vi "R6_0.vi"(1 "input variable":dbl[](array[numeric])) -> (0 "output variable":dbl[][](array[numeric]))   [LabVIEW 2018]
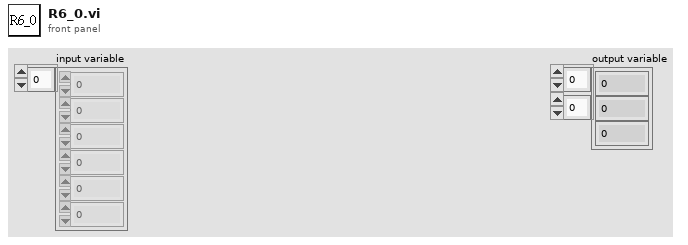
[diagram p1: front panel]
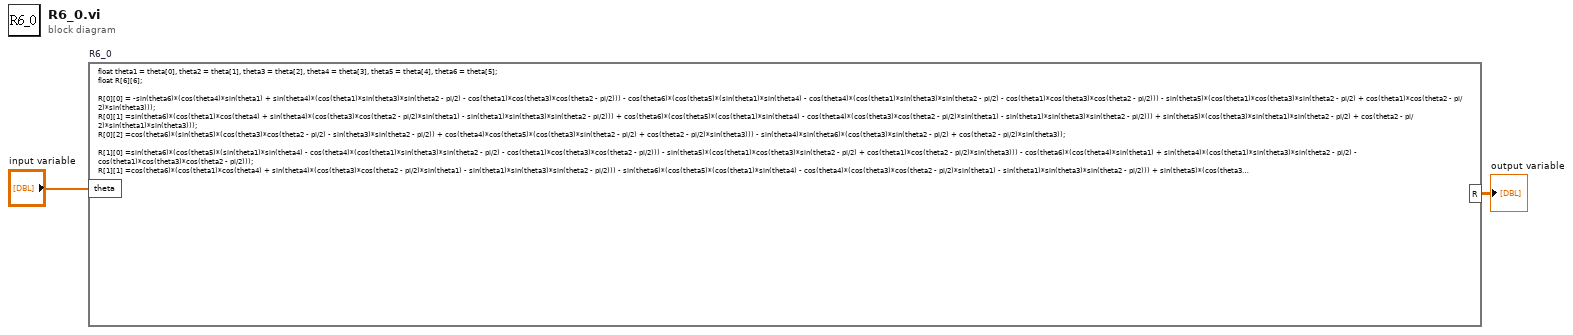
[diagram p0: block diagram]
diagram:
  n1 = formula code="float theta1 = theta[0], theta2 = theta[1], theta3 = theta[2], theta4 = theta[3], theta5 = theta[4], theta6 = theta[5];\nfloat R[6][6];\n\nR[0][0] = -sin(theta6)*(cos(theta4)*sin(theta1) + sin(theta4)*(cos(theta1)*sin(theta3)*sin(theta2 - pi/2) - cos(theta1)*cos(theta3)*cos(theta2 - pi/2))) - cos(theta6)*(cos(theta5)*(sin(theta1)*sin(theta4) - cos(theta4)*(cos(theta1)*sin(theta3)*sin(theta2 - pi/2) - cos(theta1)*cos(theta3)*cos(theta2 - pi/2))) - sin(theta5)*(cos(theta1)*cos(theta3)*sin(theta2 - pi/2) + cos(theta1)*cos(theta2 - pi/2)*sin(theta3)));\nR[0][1] =sin(theta6)*(cos(theta1)*cos(theta4) + sin(theta4)*(cos(theta3)*cos(theta2 - pi/2)*sin(theta1) - sin(theta1)*sin(theta3)*sin(theta2 - pi/2))) + cos(theta6)*(cos(theta5)*(cos(theta1)*sin(theta4) - cos(theta4)*(cos(theta3)*cos(theta2 - pi/2)*sin(theta1) - sin(theta1)*sin(theta3)*sin(theta2 - pi/2))) + sin(theta5)*(cos(theta3)*sin(theta1)*sin(theta2 - pi/2) + cos(theta2 - pi/2)*sin(theta1)*sin(theta3)));\nR[0][2] =cos(theta6)*(sin(theta5)*(cos(theta3)*cos(theta2 - pi/2) - sin(theta3)*sin(theta2 - pi/2)) + cos(theta4)*cos(theta5)*(cos(theta3)*sin(theta2 - pi/2) + cos(theta2 - pi/2)*sin(theta3))) - sin(theta4)*sin(theta6)*(cos(theta3)*sin(theta2 - pi/2) + cos(theta2 - pi/2)*sin(theta3));\n\nR[1][0] =sin(theta6)*(cos(theta5)*(sin(theta1)*sin(theta4) - cos(theta4)*(cos(theta1)*sin(theta3)*sin(theta2 - pi/2) - cos(theta1)*cos(theta3)*cos(theta2 - pi/2))) - sin(theta5)*(cos(theta1)*cos(theta3)*sin(theta2 - pi/2) + cos(theta1)*cos(theta2 - pi/2)*sin(theta3))) - cos(theta6)*(cos(theta4)*sin(theta1) + sin(theta4)*(cos(theta1)*sin(theta3)*sin(theta2 - pi/2) - cos(theta1)*cos(theta3)*cos(theta2 - pi/2)));\nR[1][1] =cos(theta6)*(cos(theta1)*cos(theta4) + sin(theta4)*(cos(theta3)*cos(theta2 - pi/2)*sin(theta1) - sin(theta1)*sin(theta3)*sin(theta2 - pi/2))) - sin(theta6)*(cos(theta5)*(cos(theta1)*sin(theta4) - cos(theta4)*(cos(theta3)*cos(theta2 - pi/2)*sin(theta1) - sin(theta1)*sin(theta3)*sin(theta2 - pi/2))) + sin(theta5)*(cos(theta3)*sin(theta1)*sin(theta2 - pi/2) + cos(theta2 - pi/2)*sin(theta1)*sin(theta3)));\nR[1][2] =-sin(theta6)*(sin(theta5)*(cos(theta3)*cos(theta2 - pi/2) - sin(theta3)*sin(theta2 - pi/2)) + cos(theta4)*cos(theta5)*(cos(theta3)*sin(theta2 - pi/2) + cos(theta2 - pi/2)*sin(theta3))) - cos(theta6)*sin(theta4)*(cos(theta3)*sin(theta2 - pi/2) + cos(theta2 - pi/2)*sin(theta3));\n\nR[2][0] =-sin(theta5)*(sin(theta1)*sin(theta4) - cos(theta4)*(cos(theta1)*sin(theta3)*sin(theta2 - pi/2) - cos(theta1)*cos(theta3)*cos(theta2 - pi/2))) - cos(theta5)*(cos(theta1)*cos(theta3)*sin(theta2 - pi/2) + cos(theta1)*cos(theta2 - pi/2)*sin(theta3));\nR[2][1] =sin(theta5)*(cos(theta1)*sin(theta4) - cos(theta4)*(cos(theta3)*cos(theta2 - pi/2)*sin(theta1) - sin(theta1)*sin(theta3)*sin(theta2 - pi/2))) - cos(theta5)*(cos(theta3)*sin(theta1)*sin(theta2 - pi/2) + cos(theta2 - pi/2)*sin(theta1)*sin(theta3));\nR[2][2] =cos(theta4)*sin(theta5)*(cos(theta3)*sin(theta2 - pi/2) + cos(theta2 - pi/2)*sin(theta3)) - cos(theta5)*(cos(theta3)*cos(theta2 - pi/2) - sin(theta3)*sin(theta2 - pi/2));" "R6_0"("theta"="input variable") -> ("R"=→"output variable":dbl[][])
